vi "Filtri acquisizioni in tabella prove.vi"() -> ()   [LabVIEW 2016]
uses:
  <vilib>/Utility/file.llb/Read Delimited Spreadsheet (string).vi
  <vilib>/Utility/file.llb/Write Delimited Spreadsheet (string).vi
  Global percorso impostazioni.vi
panel:
  in  "ORDINE COLONNE":i32(listbox)
  in  "reinizializza":bool
  in  "Save Button":bool
  in  "stop":bool
  in  "Array":T1(array[cluster]) {"Medie RT" min=-1 max=100; "decimali" min=-1 max=5}
  in  "TIPO COLLEGAMENTO":u16(ring) items=["3fase3fili", "3fase6fili", "monofase"]
  # "PROVE"
  # "QH"
  # "RES.FREDDO"
  # "TERMICA"
  # "NPSH"
  # "INCERTEZZA"
  # "GRANDEZZA"
  # "seleziona\ntipo collegamento"
  # "nota: -1 sul campo \"decimali\" significa che\ni decimali della grandezza in questione\nnon vengono gestiti. Utilizzare -1 per le \ngrandezze che non sono valori numerici\nad esempio tempo[h:m:s]"
  # "CONDIZIONI OBBLIGATORIE:\n\nI seguenti campi:\n\n-Banco\n-Anno\n-Numero\n-N°tabella\n-Misura\n-Tipo prova\n-Progressivo Acq\n\ndevono avere decimali=0 ed\nessere salvati per tutte le prove\n\nil campo\n\n-tempo[h:m:s]\n\ndeve avere decimali=-1"
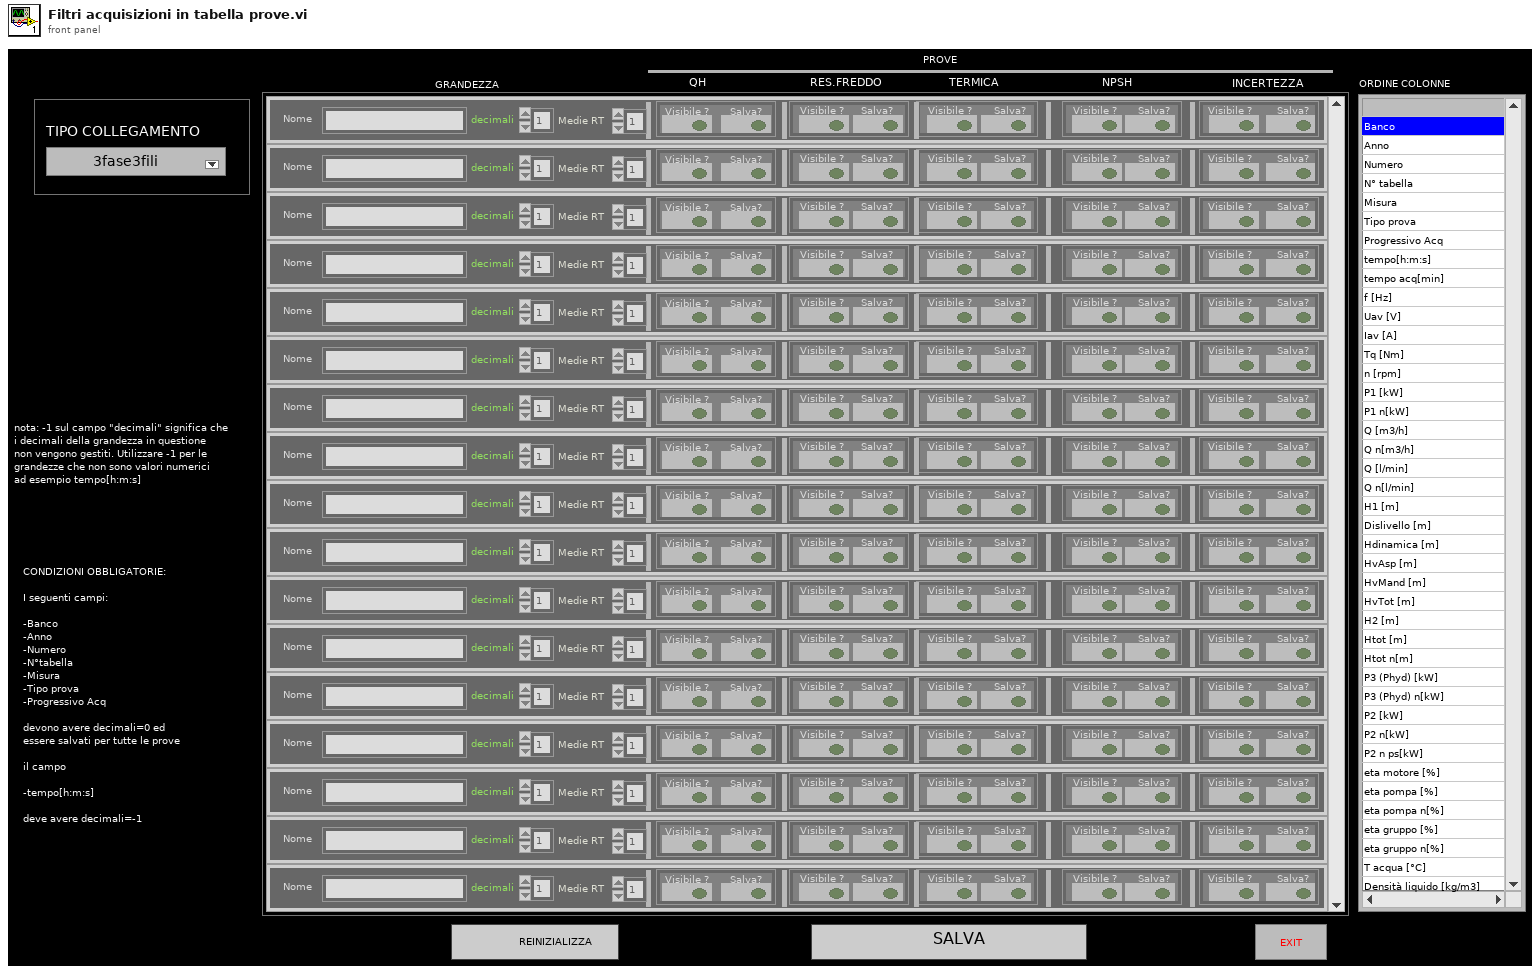
[diagram p1: front panel]
types:
  T1 = cluster{"Nome":string, "QH":cluster{"Visibile ?":bool, "Salva?":bool}, "FREDDO":cluster{"Visibile ?":bool, "Salva?":bool}, "TERMICA":cluster{"Visibile ?":bool, "Salva?":bool}, "NPSH":cluster{"Visibile ?":bool, "Salva?":bool}, "MEI":cluster{"Visibile ?":bool, "Salva?":bool}, "decimali":i8, "Medie RT":i8}[]
  T2 = cluster{"Nome":string, "QH":cluster{"Visibile ?":bool, "Salva?":bool}, "FREDDO":cluster{"Visibile ?":bool, "Salva?":bool}, "TERMICA":cluster{"Visibile ?":bool, "Salva?":bool}, "NPSH":cluster{"Visibile ?":bool, "Salva?":bool}, "MEI":cluster{"Visibile ?":bool, "Salva?":bool}, "decimali":i8, "Medie RT":i8}
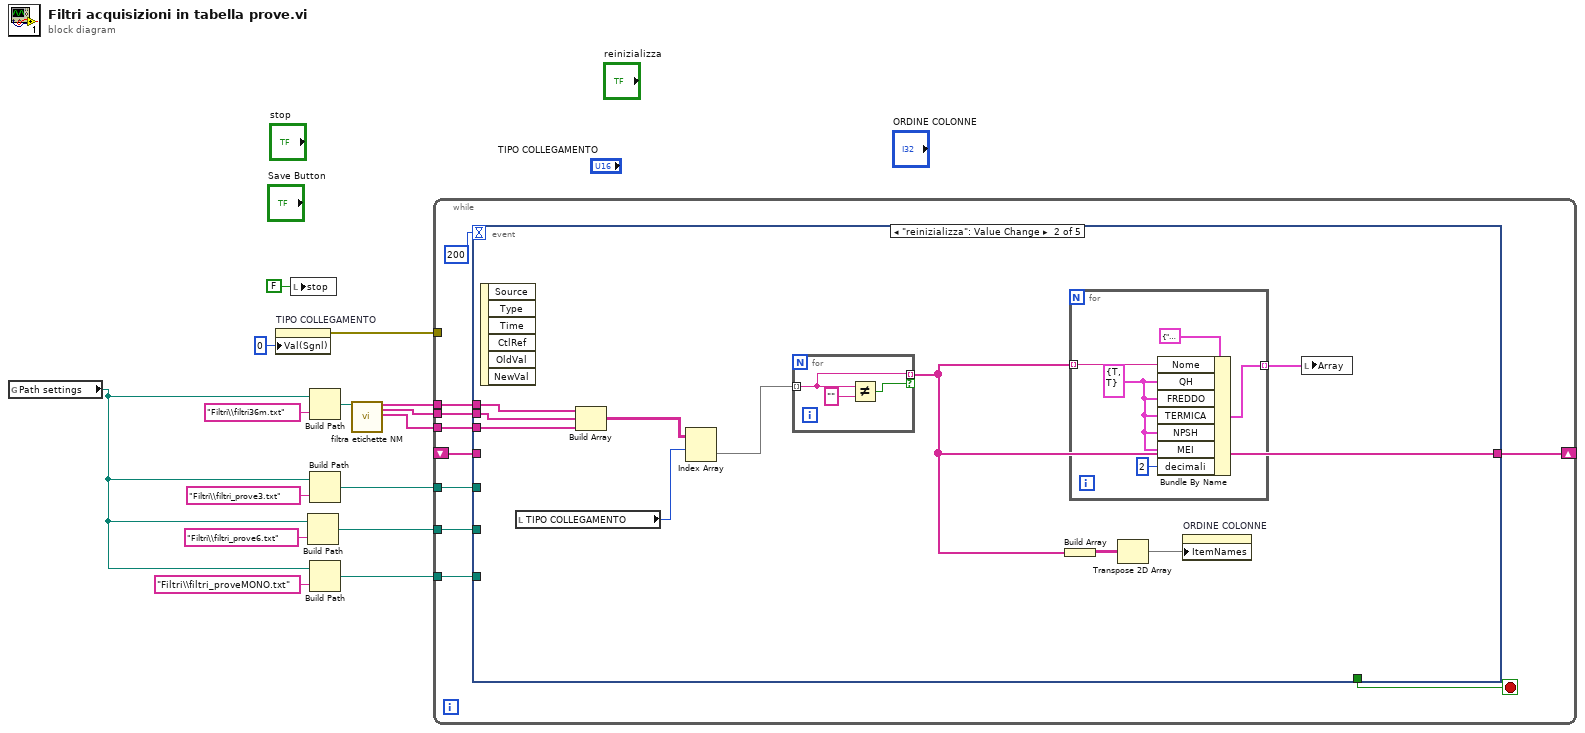
[diagram p0: block diagram]
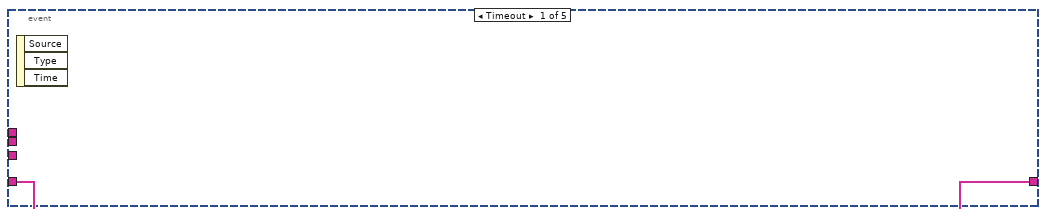
[diagram p2: hidden frame]
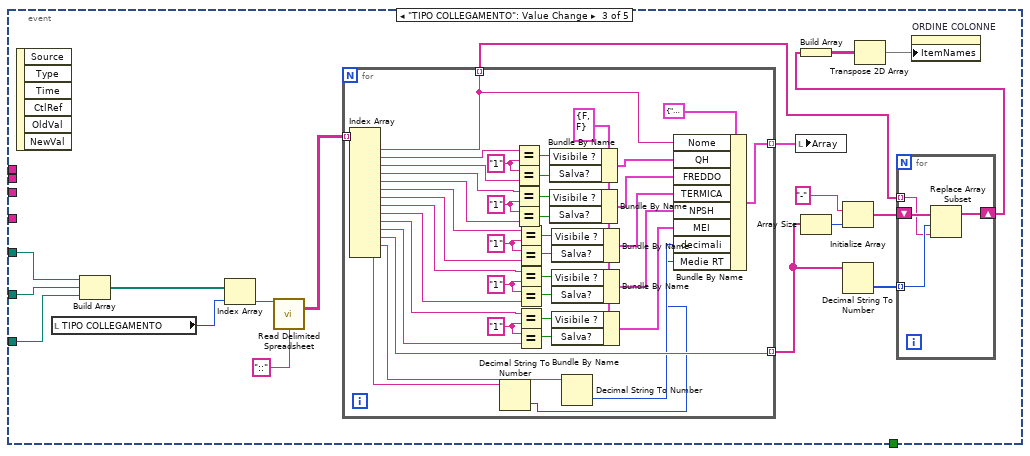
[diagram p3: hidden frame]
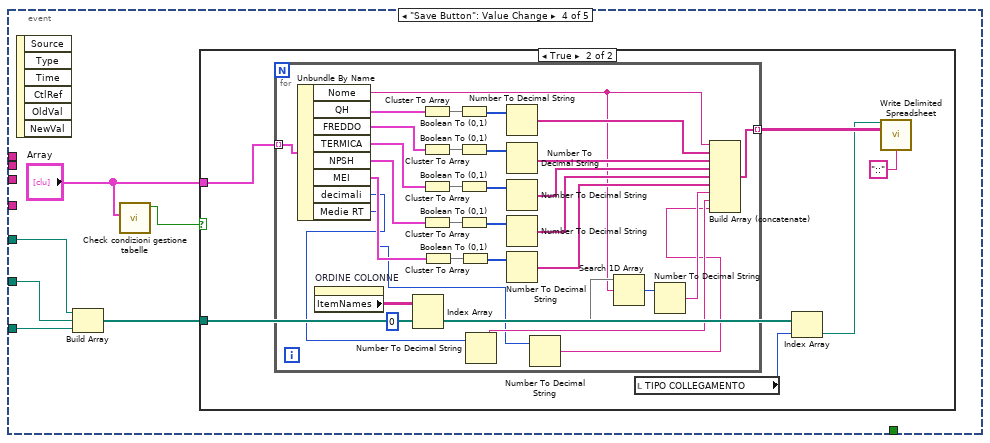
[diagram p4: hidden frame]
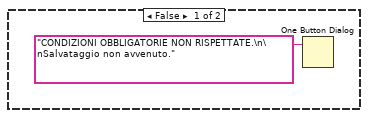
[diagram p5: hidden frame]
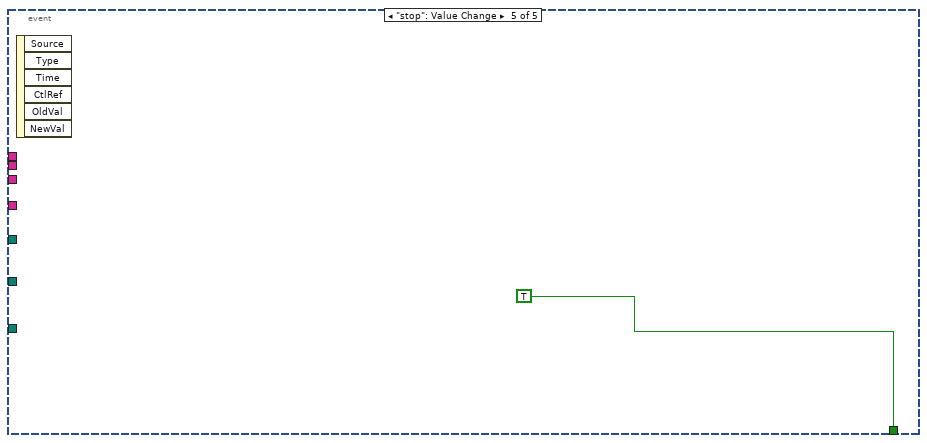
[diagram p6: hidden frame]
diagram:
  n1 = global read "Global percorso impostazioni.vi" "Path settings"() -> (w1:path)
  n2 = property on="TIPO COLLEGAMENTO" class="Ring (strict)"("Val(Sgnl)"=u16 0 ("Value (Signaling)")) -> (error out=w2:errorcluster)  [unwired: 2 in, 1 out]
  n3 = local write "stop"(FALSE ("stop")) -> ()
  n4 = Build Path(base path=w1, name or relative path="Filtri\\filtri_prove6.txt") -> (appended path=w6:path)
  n5 = Build Path(base path=w1, name or relative path="Filtri\\filtri36m.txt") -> (appended path=w14:path)
  n6 = Build Path(base path=w1, name or relative path="Filtri\\filtri_prove3.txt") -> (appended path=w7:path)
  n7 = Build Path(base path=w1, name or relative path="Filtri\\filtri_proveMONO.txt") -> (appended path=w5:path)
  n8 = call "filtra etichette NM.vi"("File filtri path"=w14) -> ("Array 3ph3ch"=w13:string[], "Array 3ph6ch"=w12:string[], "Array 1ph"=w11:string[])  [unwired: 11 in, 5 out]
  n9 = while {
    tunnel: w13 -> [w25]
    tunnel: w12 -> [w24]
    tunnel: w11 -> [w23]
    shift-right: [w22] -> _
    shift-left: _ -> [w21]
    tunnel: w7 -> [w19]
    tunnel: w6 -> [w18]
    tunnel: w5 -> [w17]
    tunnel: w2 -> [_]
    stop <- w20 stop-if-true
    n10 = event shown="[1] \"reinizializza\": Value Change" {
      selector: _ -> [_ _ _ _ _]
      dyn-events: _ -> [_ _ _ _ _]
      timeout: 200 -> [_ _ _ _ _]
      tunnel: w25 -> [_ w35 _ _ _]
      tunnel: w24 -> [_ w34 _ _ _]
      tunnel: w23 -> [_ w33 _ _ _]
      tunnel: [w26 w29 _ _ _] -> w22
      tunnel: w21 -> [w26 _ _ _ _]
      tunnel: [_ _ _ _ TRUE] -> w20
      tunnel: w19 -> [_ _ w61 w112 _]
      tunnel: w18 -> [_ _ w60 w111 _]
      tunnel: w17 -> [_ _ w59 w110 _]
      event Timeout {
        n11 = event-data() -> ()  [unwired: 1 in, 3 out]
      }
      event "reinizializza": Value Change {
        n12 = event-data() -> ()  [unwired: 1 in, 6 out]
        n13 = local read "TIPO COLLEGAMENTO"() -> (w30:u16)
        n14 = Build Array(w35, w34, w33) -> (w36:string[][])
        n15 = Index Array(array=w36, index (row)=w30) -> (element=w32:string[])  [unwired: 1 in]
        n16 = for {
          tunnel: w32 -> [w43] mode=indexing
          tunnel: [w43] -> w29 mode=indexing if=w42
          n17 = Not Equal?(x=w43, y="") -> (x != y?=w42:bool)
        }
        n18 = Build Array(w29) -> (w28:string[][])
        n19 = for {
          tunnel: w29 -> [w41] mode=indexing
          tunnel: [w40] -> w31 mode=indexing
          w39 = cluster{"Visibile ?":bool, "Salva?":bool} {"Visibile ?"=TRUE, "Salva?"=TRUE} ("QH")
          n20 = Bundle By Name(cluster=T2 {"Nome"="Banco", "QH"={"Visibile ?"=FALSE, "Salva?"=TRUE}, "FREDDO"={"Visibile ?"=FALSE, "Salva?"=TRUE}, "TERMICA"={"Visibile ?"=FALSE, "Salva?"=TRUE}, "NPSH"={"Visibile ?"=FALSE, "Salva?"=TRUE}, "MEI"={"Visibile ?"=TRUE, "Salva?"=TRUE}, "decimali"=0, "Medie RT"=1} ("Cluster"), "Nome"=w41, "QH"=w39, "FREDDO"=w39, "TERMICA"=w39, "NPSH"=w39, "MEI"=w39, "decimali"=i8 2) -> (w40:T2)
        }
        n21 = Transpose 2D Array(2D array=w28) -> (transposed array=w27:string[][])
        n22 = property on="ORDINE COLONNE" class="MCListbox (strict)"("ItemNames"=w27) -> ()  [unwired: 2 in, 2 out]
        n23 = local write "Array"(w31) -> ()
      }
      event "TIPO COLLEGAMENTO": Value Change {
        n24 = event-data() -> ()  [unwired: 1 in, 6 out]
        n25 = local read "TIPO COLLEGAMENTO"() -> (w58:u16)
        n26 = Build Array(w61, w60, w59) -> (w62:path[])
        n27 = Index Array(array=w62, index=w58) -> (element=w57:path)
        n28 = call-poly <vilib>:"Read Delimited Spreadsheet.vi"("file path (dialog if empty)"=w57, "delimiter (\\t)"="::" ("delimiter (\\t)")) -> ("all rows"=w55:string[][])  [unwired: 8 in, 5 out]
        n29 = for {
          tunnel: [w106] -> w45 mode=indexing
          tunnel: w55 -> [w105] mode=indexing
          tunnel: [w73] -> w49 mode=indexing
          tunnel: [w72] -> w52 mode=indexing
          w79 = "1" ("y")
          w91 = "1" ("y")
          w90 = "1" ("y")
          w99 = "1" ("y")
          w100 = "1" ("y")
          w77 = cluster{"Visibile ?":bool, "Salva?":bool} {"Visibile ?"=FALSE, "Salva?"=FALSE} ("QH")
          n30 = Index Array(array=w105) -> (element #1=w73:string, element #2=w103:string, element #3=w101:string, element #4=w96:string, element #5=w95:string, element #6=w88:string, element #7=w87:string, element #8=w86:string, element #9=w85:string, element #10=w76:string, element #11=w75:string, element #12=w72:string, element #13=w71:string, element #14=w68:string)  [unwired: 14 in]
          n31 = Decimal String To Number(string=w68) -> (number=w67:i32)  [unwired: 2 in, 1 out]
          n32 = Equal?(x=w103, y=w100) -> (x = y?=w104:bool)
          n33 = Equal?(x=w100, y=w101) -> (x = y?=w102:bool)
          n34 = Equal?(x=w96, y=w99) -> (x = y?=w97:bool)
          n35 = Equal?(x=w99, y=w95) -> (x = y?=w98:bool)
          n36 = Equal?(x=w88, y=w90) -> (x = y?=w89:bool)
          n37 = Equal?(x=w90, y=w87) -> (x = y?=w84:bool)
          n38 = Equal?(x=w86, y=w91) -> (x = y?=w92:bool)
          n39 = Equal?(x=w91, y=w85) -> (x = y?=w83:bool)
          n40 = Equal?(x=w76, y=w79) -> (x = y?=w78:bool)
          n41 = Equal?(x=w79, y=w75) -> (x = y?=w80:bool)
          n42 = Bundle By Name(cluster=w77, "Visibile ?"=w104, "Salva?"=w102) -> (w94:cluster{"Visibile ?":bool, "Salva?":bool})
          n43 = Bundle By Name(cluster=w77, "Visibile ?"=w97, "Salva?"=w98) -> (w93:cluster{"Visibile ?":bool, "Salva?":bool})
          n44 = Bundle By Name(cluster=w77, "Visibile ?"=w89, "Salva?"=w84) -> (w82:cluster{"Visibile ?":bool, "Salva?":bool})
          n45 = Bundle By Name(cluster=w77, "Visibile ?"=w92, "Salva?"=w83) -> (w81:cluster{"Visibile ?":bool, "Salva?":bool})
          n46 = Bundle By Name(cluster=w77, "Visibile ?"=w78, "Salva?"=w80) -> (w74:cluster{"Visibile ?":bool, "Salva?":bool})
          n47 = Decimal String To Number(string=w71) -> (number=w70:i32)  [unwired: 2 in, 1 out]
          n48 = Bundle By Name(cluster=T2 {"Nome"="Banco", "QH"={"Visibile ?"=FALSE, "Salva?"=TRUE}, "FREDDO"={"Visibile ?"=FALSE, "Salva?"=TRUE}, "TERMICA"={"Visibile ?"=FALSE, "Salva?"=TRUE}, "NPSH"={"Visibile ?"=FALSE, "Salva?"=TRUE}, "MEI"={"Visibile ?"=TRUE, "Salva?"=TRUE}, "decimali"=0, "Medie RT"=1} ("Cluster"), "Nome"=w73, "QH"=w94, "FREDDO"=w93, "TERMICA"=w82, "NPSH"=w81, "MEI"=w74, "decimali"=w70, "Medie RT"=w67) -> (w106:T2)
        }
        n49 = local write "Array"(w45) -> ()
        n50 = Array Size(array=w52) -> (size(s)=w51:i32)
        n51 = Initialize Array("-", w51) -> (w48:string[])
        n52 = Decimal String To Number(string=w52) -> (number=w50:i32[])  [unwired: 2 in, 1 out]
        n53 = for {
          tunnel: w50 -> [w65] mode=indexing
          tunnel: w49 -> [w64] mode=indexing
          shift-right: [w63] -> w47
          shift-left: w48 -> [w66]
          n54 = Replace Array Subset(array=w66, new element=w64, index=w65) -> (w63:string[])
        }
        n55 = Build Array(w47) -> (w54:string[][])
        n56 = Transpose 2D Array(2D array=w54) -> (transposed array=w46:string[][])
        n57 = property on="ORDINE COLONNE" class="MCListbox (strict)"("ItemNames"=w46) -> ()  [unwired: 2 in, 2 out]
      }
      event "Save Button": Value Change {
        n58 = event-data() -> ()  [unwired: 1 in, 6 out]
        n59 = Build Array(w112, w111, w110) -> (w109:path[])
        n60 = call "Check condizioni gestione tabelle.vi"("Array 2"="Array") -> ("condizioni ok"=w108:bool)  [unwired: 10 in]
        n61 = case shown="True" w108 {
          tunnel: w109 -> [_ w117]
          tunnel: "Array" -> [_ w114]
          frame False {
            n62 = One Button Dialog(message="CONDIZIONI OBBLIGATORIE NON RISPETTATE.\n\nSalvataggio non avvenuto.") -> ()  [unwired: 1 in, 1 out]
          }
          frame True {
            n63 = for {
              tunnel: w114 -> [w151] mode=indexing
              tunnel: [w150] -> w119 mode=indexing
              n64 = Unbundle By Name(w151) -> ("Nome"=w126:string, "QH"=w149:cluster{"Visibile ?":bool, "Salva?":bool}, "FREDDO"=w140:cluster{"Visibile ?":bool, "Salva?":bool}, "TERMICA"=w139:cluster{"Visibile ?":bool, "Salva?":bool}, "NPSH"=w138:cluster{"Visibile ?":bool, "Salva?":bool}, "MEI"=w136:cluster{"Visibile ?":bool, "Salva?":bool}, "decimali"=w123:i8, "Medie RT"=w120:i8)
              n65 = property on="ORDINE COLONNE" class="MCListbox (strict)"() -> ("ItemNames"=w129:string[][])  [unwired: 2 in, 2 out]
              n66 = Index Array(array=w129, index (col)=0 ("disabled index (col)")) -> (element=w128:string[])  [unwired: 1 in]
              n67 = Cluster To Array(cluster=w149) -> (array=w148:bool[])
              n68 = Cluster To Array(cluster=w140) -> (array=w145:bool[])
              n69 = Cluster To Array(cluster=w139) -> (array=w144:bool[])
              n70 = Cluster To Array(cluster=w138) -> (array=w141:bool[])
              n71 = Cluster To Array(cluster=w136) -> (array=w135:bool[])
              n72 = Boolean To (0,1)(Boolean=w148) -> (0, 1=w147:i16[])
              n73 = Boolean To (0,1)(Boolean=w145) -> (0, 1=w146:i16[])
              n74 = Boolean To (0,1)(Boolean=w144) -> (0, 1=w143:i16[])
              n75 = Boolean To (0,1)(Boolean=w141) -> (0, 1=w142:i16[])
              n76 = Boolean To (0,1)(Boolean=w135) -> (0, 1=w137:i16[])
              n77 = Number To Decimal String(number=w123) -> (decimal integer string=w122:string)  [unwired: 1 in]
              n78 = Number To Decimal String(number=w147) -> (decimal integer string=w134:string[])  [unwired: 1 in]
              n79 = Number To Decimal String(number=w146) -> (decimal integer string=w133:string[])  [unwired: 1 in]
              n80 = Number To Decimal String(number=w143) -> (decimal integer string=w132:string[])  [unwired: 1 in]
              n81 = Number To Decimal String(number=w142) -> (decimal integer string=w131:string[])  [unwired: 1 in]
              n82 = Number To Decimal String(number=w137) -> (decimal integer string=w130:string[])  [unwired: 1 in]
              n83 = Number To Decimal String(number=w120) -> (decimal integer string=w121:string)  [unwired: 1 in]
              n84 = Search 1D Array(1D array=w128, element=w126) -> (index of element=w125:i32)  [unwired: 1 in]
              n85 = Number To Decimal String(number=w125) -> (decimal integer string=w124:string)  [unwired: 1 in]
              n86 = Build Array (concatenate)(w126, w134, w133, w132, w131, w130, w124, w122, w121) -> (w150:string[])
            }
            n87 = local read "TIPO COLLEGAMENTO"() -> (w116:u16)
            n88 = Index Array(array=w117, index=w116) -> (element=w115:path)
            n89 = call-poly <vilib>:"Write Delimited Spreadsheet.vi"("file path (dialog if empty)"=w115, "2D data"=w119, "delimiter (\\t)"="::" ("delimiter (\\t)")) -> ()  [unwired: 11 in, 2 out]
          }
        }
      }
      event "stop": Value Change {
        n90 = event-data() -> ()  [unwired: 1 in, 6 out]
      }
    }
  }
